vi "Config Path--constant.vi"() -> (3 "Config Path":path)   [LabVIEW 2023, in "VI Properties Editor.lvlib"]
doc: "Outputs the path to the main config file of the tool."
uses:
  VI Properties Editor.lvlib
  <vilib>/Utility/sysdir.llb/System Directory Type.ctl
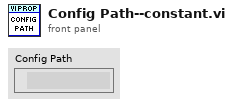
[diagram p1: front panel]
types:
  T1 = typedef "System Directory Type.ctl" = i32
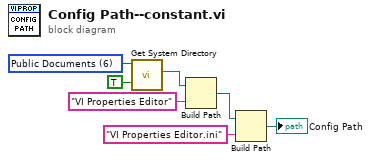
[diagram p0: block diagram]
diagram:
  w2 = T1 6 items=["User Home"=0, "User Desktop"=1, "User Documents"=2, "User Application Data"=3, "User Preferences"=4, "User Temporary"=5, "Public Documents"=6, "Public Application Data"=7, "Public Preferences"=8, "Public Cache"=13, "System Core Libraries"=9, "System Installed Libraries"=10, "Application Files"=11, "Boot Volume Root"=12] ("system directory type")
  n1 = call <vilib>:"Get System Directory.vi"("create directory if not found? (F)"=TRUE, "system directory type"=w2) -> ("system directory"=w4:path)  [unwired: 9 in]
  n2 = Build Path(base path=w4, name or relative path="VI Properties Editor") -> (appended path=w1:path)
  n3 = Build Path(base path=w1, name or relative path="VI Properties Editor.ini") -> (appended path=→"Config Path":path)
